vi "Part 1.vi"(11 "Input":string) -> (3 "Output":i64)   [LabVIEW 2021]
uses:
  <userlib>/_OpenG.lib/string/string.llb/Convert EOLs (String)__ogtk.vi
  <vilib>/Analysis/NI_AALPro.lvlib
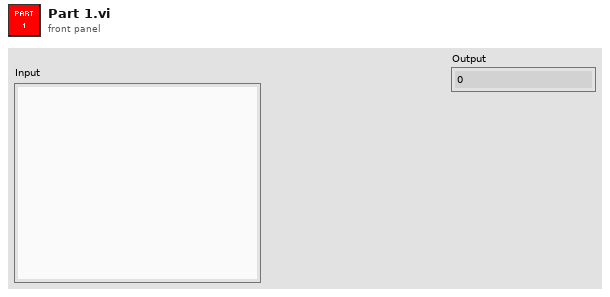
[diagram p1: front panel]
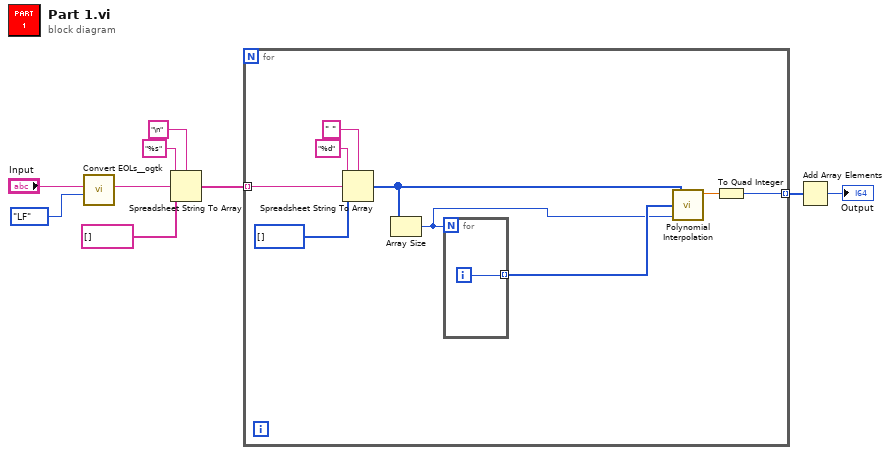
[diagram p0: block diagram]
diagram:
  n1 = call-poly <userlib>:"Convert EOLs__ogtk.vi"("Convert to:"=enum16{"CR", "LF", "CRLF"}."LF", "String in"="Input") -> ("String out"=w5:string)  [unwired: 9 in]
  n2 = Spreadsheet String To Array(delimiter (Tab)="\n", format string="%s", spreadsheet string=w5, array type (2D Dbl)=string[] []) -> (array=w3:string[])
  n3 = for {
    tunnel: w3 -> [w15] mode=indexing
    tunnel: [w10] -> w2 mode=indexing
    n4 = Spreadsheet String To Array(delimiter (Tab)=" ", format string="%d", spreadsheet string=w15, array type (2D Dbl)=i32[] []) -> (array=w13:i32[])
    n5 = Array Size(array=w13) -> (size(s)=w12:i32)
    n6 = for {
      N: w12 -> [_]
      tunnel: [w19] -> w14 mode=indexing
      i -> [w19]
    }
    n7 = call <vilib>:"Polynomial Interpolation.vi"("x value"=w12, "X"=w14, "Y"=w13) -> ("interpolation value"=w11:dbl)  [unwired: 2 out]
    n8 = To Quad Integer(1:w11) -> (0:w10:i64)
  }
  n9 = Add Array Elements(numeric array=w2) -> (sum=→"Output":i64)
